vi "pos_displayunit2encoder.vi"(8 "error in (no error)":errorcluster, 10 "pos in display unit":dbl, 11 "Motor in":refnum<class "Motor.lvclass">) -> (0 "error out":errorcluster, 2 "encoder (unit)":dbl, 3 "Motor out":refnum<class "Motor.lvclass">)   [LabVIEW 2016, in "Hardware.lvlib" / "Motor.lvlib" / "Motor.lvclass"]
uses:
  <userlib>/Common Components/Hardware/Motor/Motor/Motor.lvclass
  <userlib>/Common Components/Hardware/Motor/Motor/Motor.lvclass/Motor.ctl
  <userlib>/Common Components/Hardware/Motor/Motor/Accessor/Read unit mode.vi
  <userlib>/Common Components/Hardware/Motor/Motor/Accessor/Read motor pulses per revolution.vi
  <userlib>/Common Components/Hardware/Motor/Motor/Accessor/Read display units per motor rev.vi
  <userlib>/Common Components/Hardware/Motor/Motor/Accessor/Read encoder units ratio.vi
  <userlib>/Common Components/Hardware/Motor/Motor/Accessor/Read encoder type.vi
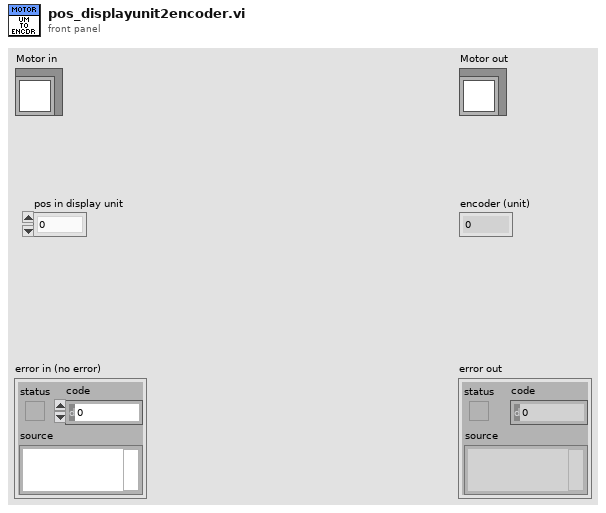
[diagram p1: front panel]
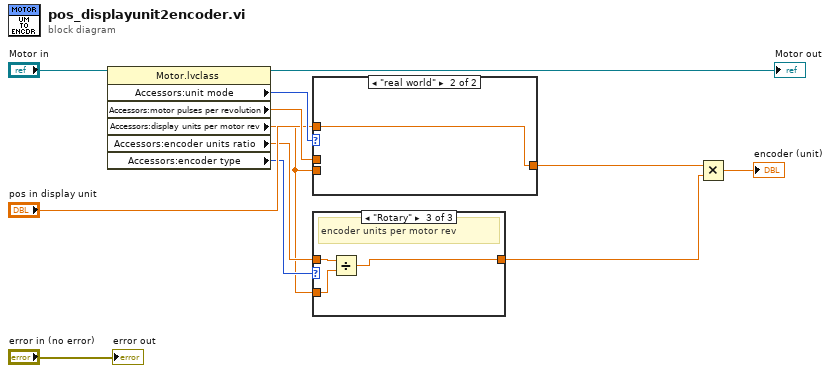
[diagram p0: block diagram]
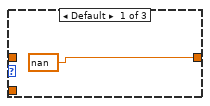
[diagram p2: hidden frame]
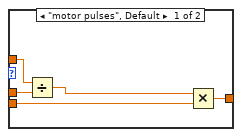
[diagram p4: hidden frame]
diagram:
  n1 = property class="Motor.lvclass"(reference="Motor in") -> (reference out=→"Motor out":refnum<class "Motor.lvclass">, "Accessors:unit mode"=w9:enum16{"motor pulses", "real world"}, "Accessors:motor pulses per revolution"=w8:dbl, "Accessors:display units per motor rev"=w1:dbl, "Accessors:encoder units ratio"=w3:dbl, "Accessors:encoder type"=w4:enum16{"Linear", "Rotary"})  [unwired: 1 in, 1 out]
  n2 = case shown="\"real world\"" w9 {
    tunnel: w8 -> [w16 _]
    tunnel: w1 -> [w14 _]
    tunnel: "pos in display unit" -> [w17 w18]
    tunnel: [w13 w18] -> w6
    frame "motor pulses", Default {
      n3 = Divide(x=w17, y=w16) -> (x/y=w15:dbl)
      n4 = Multiply(x=w15, y=w14) -> (x*y=w13:dbl)
    }
    frame "real world" {
    }
  }
  n5 = case shown="\"Rotary\"" w4 {
    tunnel: w3 -> [_ w20 w23]
    tunnel: [nan ("Accessors:encoder units ratio") w20 w21] -> w2
    tunnel: w1 -> [_ _ w22]
    frame Default {
    }
    frame "Linear" {
      # "encoder units per display units"
    }
    frame "Rotary" {
      # "encoder units per motor rev"
      n6 = Divide(x=w23, y=w22) -> (x/y=w21:dbl)
    }
  }
  n7 = Multiply(x=w6, y=w2) -> (x*y=→"encoder (unit)":dbl)
  "error out" <- "error in (no error)"
